vi "Test OpenCVFaceDetect.vi"() -> ()   [LabVIEW 2021]
uses:
  YAFTAFModule_OpenCV_Camera/OpenCVCam/OpenCVCam.lvclass
  OpenCVFaceDetection.lvclass
  Library_UserInterface_FrontPanelControl/FrontPanelControl/FrontPanelControl.lvclass
panel:
  in  "Stop":bool
  out "2D Picture":picture
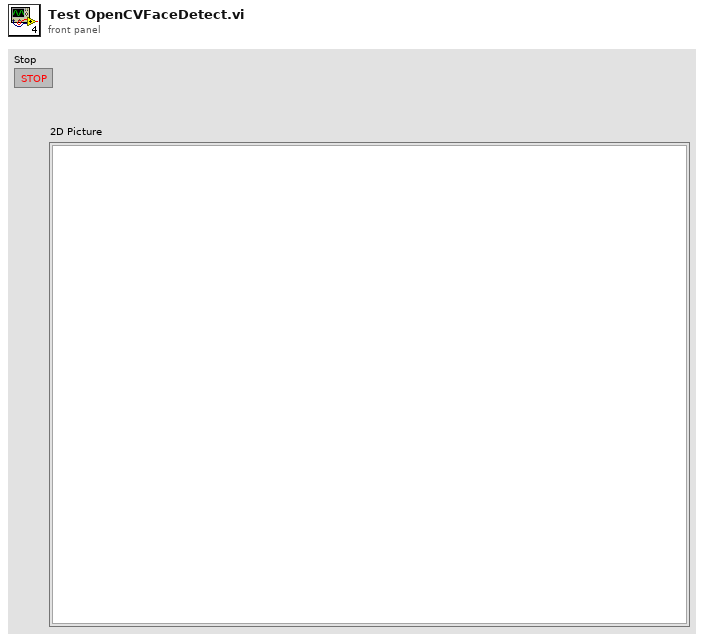
[diagram p1: front panel]
types:
  T1 = typedef "ClusterArrayConversion.lvlib/BundledArray.ctl" = cluster{"Label":string, "Object":refnum<class>, "Array":bool}
  T2 = typedef "imagedata.ctl" = cluster{"image type":i32, "image depth":i32, "image":u8[], "mask":u8[], "colors":u32[], "Rectangle":cluster{"left":i16, "top":i16, "right":i16, "bottom":i16}}
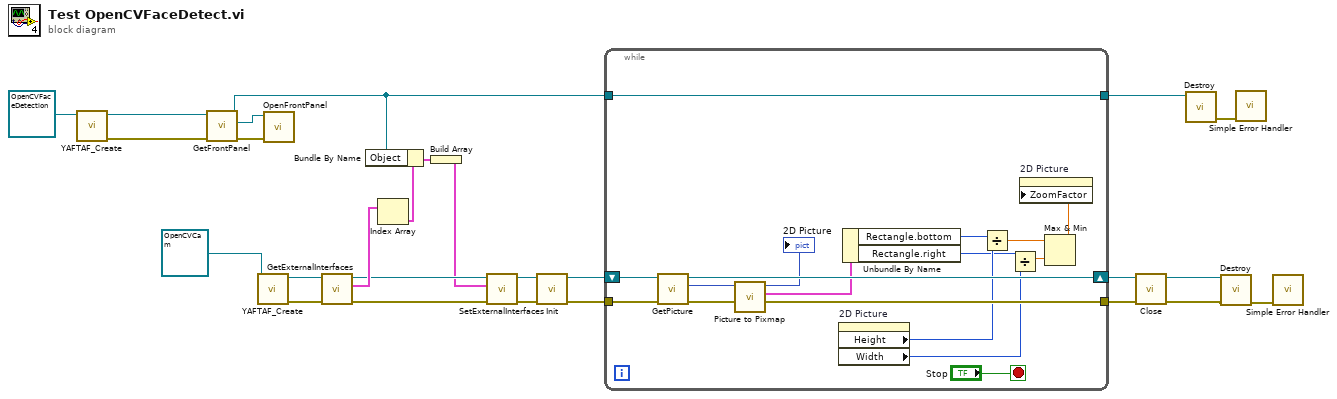
[diagram p0: block diagram]
diagram:
  n1 = call-dynamic "YAFTAF_Create.vi"("ObjectIn"=refnum<class "OpenCVFaceDetection.lvclass"> refnum ("OpenCVFaceDetection")) -> ("ErrorOut"=w19:errorcluster, "ObjectOut"=w4:refnum<class "OpenCVFaceDetection.lvclass">)  [unwired: 9 in]
  n2 = call-dynamic "GetFrontPanel.vi"("ErrorIn"=w19, "ObjectIn"=w4) -> ("ErrorOut"=w18:errorcluster, "FrontPanelControl"=w3:refnum<class "FrontPanelControl.lvclass">, "ObjectOut"=w2:refnum<class "OpenCVFaceDetection.lvclass">)  [unwired: 7 in]
  n3 = call-dynamic "YAFTAF_Create.vi"("ObjectIn"=refnum<class "OpenCVCam.lvclass"> refnum ("OpenCVCam")) -> ("ErrorOut"=w22:errorcluster, "ObjectOut"=w11:refnum<class "OpenCVCam.lvclass">)  [unwired: 9 in]
  n4 = call-dynamic "OpenFrontPanel.vi"("ErrorIn"=w18, "ObjectIn"=w3) -> ()  [unwired: 8 in, 2 out]
  n5 = call-dynamic "GetExternalInterfaces.vi"("ErrorIn"=w22, "ObjectIn"=w11) -> ("ErrorOut"=w21:errorcluster, "ExternalInterfaces"=w10:T1[], "ObjectOut"=w8:refnum<class "OpenCVCam.lvclass">)  [unwired: 7 in]
  n6 = Index Array(array=w10) -> (element=w9:T1)  [unwired: 1 in]
  n7 = Bundle By Name(cluster=w9, "Object"=w2) -> (w6:T1)
  n8 = Build Array(w6) -> (w5:T1[])
  n9 = call-dynamic "SetExternalInterfaces.vi"("ErrorIn"=w21, "ExternalInterfaces"=w5, "ObjectIn"=w8) -> ("ErrorOut"=w20:errorcluster, "ObjectOut"=w7:refnum<class "OpenCVCam.lvclass">)  [unwired: 7 in]
  n10 = call-dynamic "Init.vi"("ErrorIn"=w20, "OpenCVCamIn"=w7) -> ("ErrorOut"=w26:errorcluster, "OpenCVCamOut"=w16:refnum<class "OpenCVCam.lvclass">)  [unwired: 8 in]
  n11 = while {
    shift-right: [w39] -> w15
    shift-left: w16 -> [w40]
    tunnel: w26 -> [w42]
    tunnel: [w41] -> w25
    tunnel: [w27] -> w1
    tunnel: w2 -> [w27]
    stop <- "Stop" stop-if-true
    n12 = call-dynamic "GetPicture.vi"("ErrorIn"=w42, "OpenCVCamIn"=w40) -> ("ErrorOut"=w41:errorcluster, "2D Picture"=w37:picture, "OpenCVCamOut"=w39:refnum<class "OpenCVCam.lvclass">)  [unwired: 7 in]
    n13 = call <vilib>:"Picture to Pixmap.vi"("picture"=w37) -> ("image data"=w35:T2, "new picture"=→"2D Picture":picture)  [unwired: 9 in]
    n14 = property on="2D Picture" class="Pict"() -> ("Height"=w33:u32, "Width"=w31:u32)  [unwired: 2 in, 2 out]
    n15 = Unbundle By Name(w35) -> ("Rectangle.bottom"=w34:i16, "Rectangle.right"=w32:i16)
    n16 = Divide(x=w34, y=w33) -> (x/y=w29:dbl)
    n17 = Divide(x=w32, y=w31) -> (x/y=w30:dbl)
    n18 = Max & Min(x=w29, y=w30) -> (max(x,y)=w28:dbl)  [unwired: 1 out]
    n19 = property on="2D Picture" class="Pict"("ZoomFactor"=w28) -> ()  [unwired: 2 in, 2 out]
  }
  n20 = call-dynamic "Close.vi"("ErrorIn"=w25, "OpenCVCamIn"=w15) -> ("ErrorOut"=w24:errorcluster, "OpenCVCamOut"=w14:refnum<class "OpenCVCam.lvclass">)  [unwired: 8 in]
  n21 = call-dynamic "Destroy.vi"("ObjectIn"=w1) -> ("ErrorOut"=w17:errorcluster)  [unwired: 9 in, 1 out]
  n22 = call-dynamic "Destroy.vi"("ErrorIn"=w24, "ObjectIn"=w14) -> ("ErrorOut"=w23:errorcluster)  [unwired: 8 in, 1 out]
  n23 = call <vilib>:"Simple Error Handler.vi"("error in (no error)"=w17) -> ()  [unwired: 4 in, 5 out]
  n24 = call <vilib>:"Simple Error Handler.vi"("error in (no error)"=w23) -> ()  [unwired: 4 in, 5 out]
